vi "Vector2_Cross_Product_PN.vi"(1 "V (2D)":dbl[](array[numeric])=[0.0, 1.0], 2 "U (2D)":dbl[](array[numeric])=[1.0, 0.0]) -> (0 "U X V (2D)":dbl=1.0)   [LabVIEW 2011]
panel:
  # "Returns the z component of the usual Vector3 cross product"
  # "Paul Nathan 12/12/09"
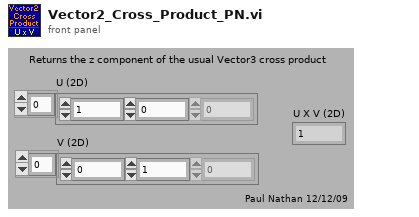
[diagram p1: front panel]
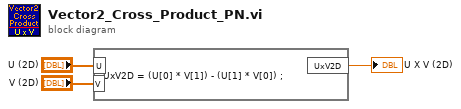
[diagram p0: block diagram]
diagram:
  n1 = formula code="UxV2D = (U[0] * V[1]) - (U[1] * V[0]) ;"("U"="U (2D)", "V"="V (2D)") -> ("UxV2D"=→"U X V (2D)":dbl)
